vi "Using string functions.vi"() -> ()   [LabVIEW 2024]
panel:
  out "result string":string
  out "replaced substring":string
  out "x .xor. y?":i32
  in  "Numeric 2":dbl
  in  "Numeric":dbl
  out "offset past match":i32
  out "after substring":string
  out "match substring":string
  out "before substring":string
  in  "offset (0)":i32
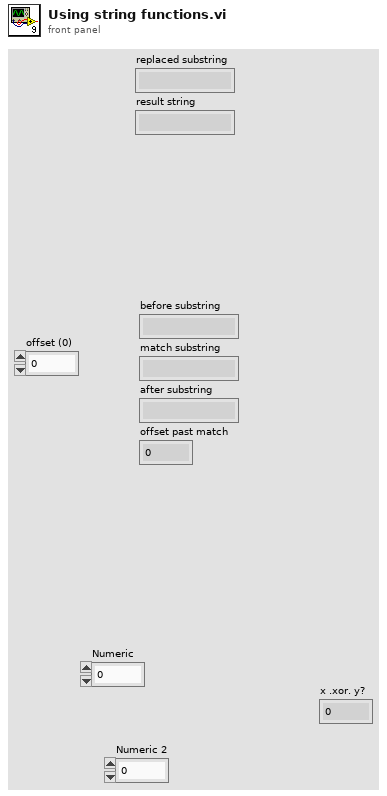
[diagram p1: front panel]
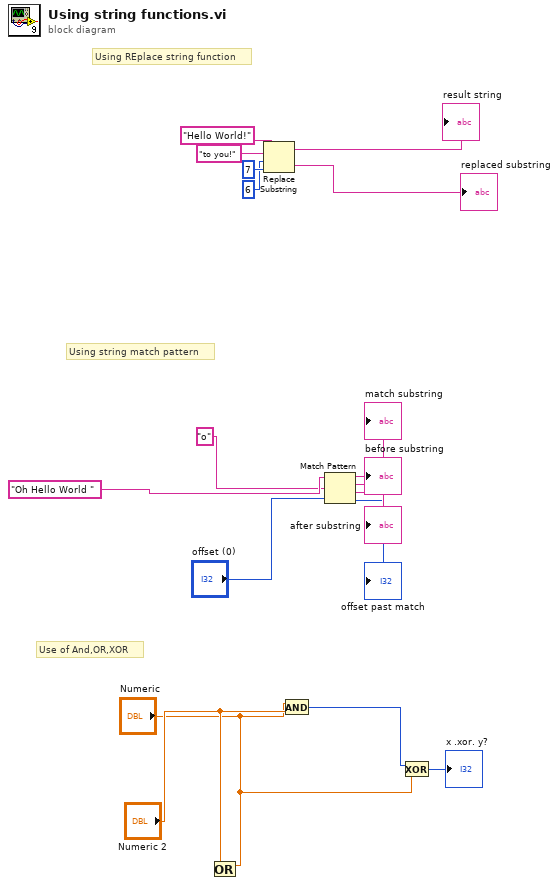
[diagram p0: block diagram]
diagram:
  # "Use of And,OR,XOR"
  # "Using REplace string function"
  # "Using string match pattern"
  n1 = Or(x="Numeric", y="Numeric 2") -> ()  [unwired: 1 out]
  n2 = Replace Substring(2:7 ("length (len. of substring)"), 3:6 ("offset (0)"), 4:"to you!" ("substring (\"\")"), 5:"Hello World!" ("string")) -> (0:→"replaced substring":string, 1:→"result string":string)
  n3 = And(x="Numeric", y="Numeric 2") -> (x .and. y?=w10:i32)
  n4 = Match Pattern(string="Oh Hello World ", regular expression="o" ("string"), offset (0)="offset (0)") -> (before substring=→"before substring":string, match substring=→"match substring":string, after substring=→"after substring":string, offset past match=→"offset past match":i32)
  n5 = Exclusive Or(1:"Numeric", 2:w10) -> (0:→"x .xor. y?":i32)
